vi "0~9顯示器.vi"() -> ()   [LabVIEW 2015]
panel:
  in  "Numeric":i32=9
  in  "Array":bool[](array[boolean])=[FALSE, FALSE, FALSE, FALSE, FALSE, FALSE, FALSE]
  out "7":bool
  out "6":bool
  out "5":bool
  out "4":bool
  out "3":bool
  out "2":bool
  out "1":bool
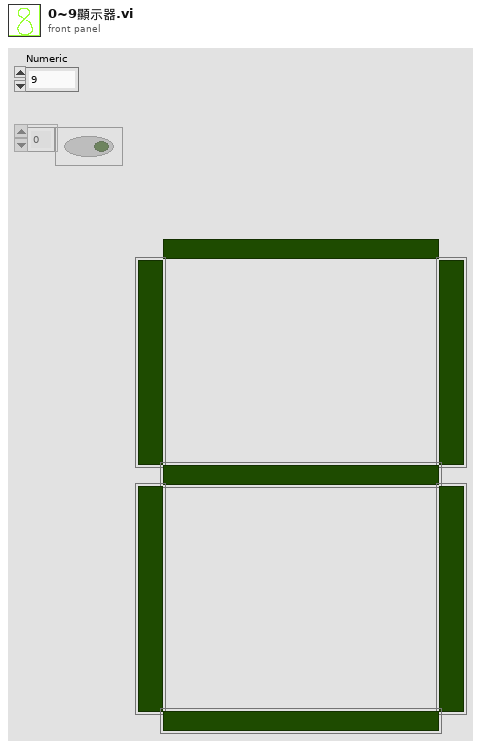
[diagram p1: front panel]
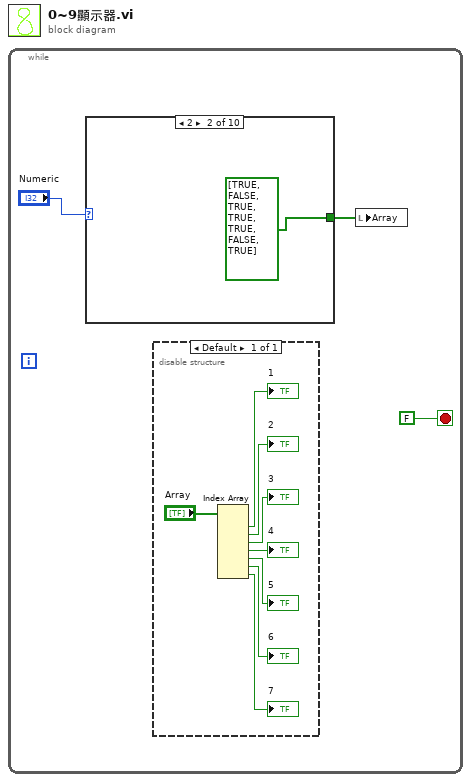
[diagram p0: block diagram]
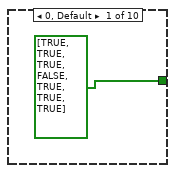
[diagram p2: hidden frame]
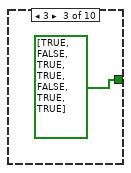
[diagram p3: hidden frame]
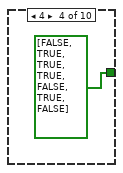
[diagram p4: hidden frame]
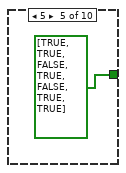
[diagram p5: hidden frame]
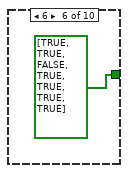
[diagram p6: hidden frame]
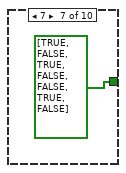
[diagram p7: hidden frame]
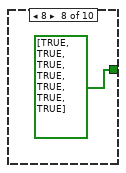
[diagram p8: hidden frame]
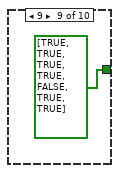
[diagram p9: hidden frame]
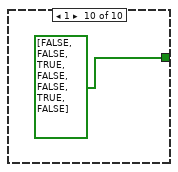
[diagram p10: hidden frame]
diagram:
  n1 = while {
    stop <- FALSE stop-if-true
    n2 = case shown="2" "Numeric" {
      tunnel: [bool[] [TRUE, TRUE, TRUE, FALSE, TRUE, TRUE, TRUE] ("Array") bool[] [TRUE, FALSE, TRUE, TRUE, TRUE, FALSE, TRUE] ("Array") bool[] [TRUE, FALSE, TRUE, TRUE, FALSE, TRUE, TRUE] ("Array") bool[] [FALSE, TRUE, TRUE, TRUE, FALSE, TRUE, FALSE] ("Array") bool[] [TRUE, TRUE, FALSE, TRUE, FALSE, TRUE, TRUE] ("Array") bool[] [TRUE, TRUE, FALSE, TRUE, TRUE, TRUE, TRUE] ("Array") bool[] [TRUE, FALSE, TRUE, FALSE, FALSE, TRUE, FALSE] ("Array") bool[] [TRUE, TRUE, TRUE, TRUE, TRUE, TRUE, TRUE] ("Array") bool[] [TRUE, TRUE, TRUE, TRUE, FALSE, TRUE, TRUE] ("Array") bool[] [FALSE, FALSE, TRUE, FALSE, FALSE, TRUE, FALSE] ("Array")] -> w2
      frame 0, Default {
      }
      frame 2 {
      }
      frame 3 {
      }
      frame 4 {
      }
      frame 5 {
      }
      frame 6 {
      }
      frame 7 {
      }
      frame 8 {
      }
      frame 9 {
      }
      frame 1 {
      }
    }
    n3 = disable-structure shown="Default" {
      frame Enabled {
        n4 = Index Array(array="Array") -> (element #1=→"1":bool, element #2=→"2":bool, element #3=→"3":bool, element #4=→"4":bool, element #5=→"5":bool, element #6=→"6":bool, element #7=→"7":bool)  [unwired: 7 in]
      }
    }
    n5 = local write "Array"(w2) -> ()
  }
